vi "GetQR_A.vi"(8 "error in":errorcluster, 10 "Image In":T2, 11 "Session In":T1) -> (0 "error out":errorcluster, 1 "QR_OK":bool, 2 "QR_CODE":string, 3 "Image Out":T2(plugin-control))   [LabVIEW 2018]
uses:
  <vilib>/vision/Image Controls.llb/IMAQ Image.ctl
  <vilib>/userdefined/High Color/IMAQdx.ctl
  <vilib>/vision/NI_Vision_Development_Module.lvlib
  <vilib>/vision/driver/NI_Vision_Acquisition_Software.lvlib
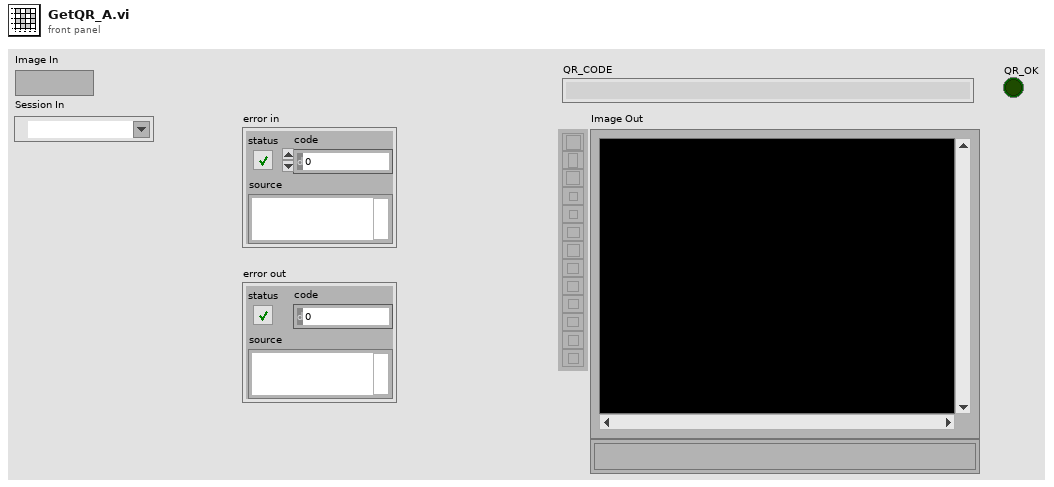
[diagram p1: front panel]
types:
  T1 = typedef "IMAQdx.ctl" = refnum<k21>
  T2 = typedef "IMAQ Image.ctl" = refnum<image>
  T3 = cluster{"Matrix Dimensions (cells)":i32, "Barcode Polarity":i32, "Mirror Mode":i32, "QR Model":i32}
  T4 = cluster{"Global Rectangle":i32[], "Contours":cluster{"ID":enum32{"External", "Internal"}, "Type":u32, "Coordinates":i32[]}[]}
  T5 = cluster{"Rotation Mode":enum32{"Unlimited", "0 Degrees", "90 Degrees", "180 Degrees", "270 Degrees"}, "Skip Location?":bool, "Edge Threshold":u32, "Demodulation Mode":i32, "Cell Sample Size":i32, "Cell Filter Mode":i32, "Skew Degrees Allowed":u32}
  T6 = typedef "QR Code Report.ctl" = cluster{"Found?":bool, "Data":string, "Bounding Box":cluster{"x":sgl, "y":sgl}[], "Errors Corrected":u32, "Dimensions (Rows/Cols)":u32, "Version":u32, "QR Model":T7, "Stream Mode":T8, "Barcode Polarity":T9, "Mirrored?":bool, "Append Stream Position":u32, "Size of Append Stream":u32, "First EAN-128 ID":i32, "First Alternate Language ID":i32, "Append Stream ID":u32, "Minimum Edge Strength":u32, "Demodulation Mode":T10, "Cell Sample Size":T11, "Cell Filter Mode":T12}
  T7 = typedef "QR Code Model Type.ctl" = i32
  T8 = typedef "QR Code Stream Mode Type.ctl" = i32
  T9 = typedef "Data Matrix Polarity.ctl" = i32
  T10 = typedef "Demodulation Mode.ctl" = i32
  T11 = typedef "Cell Sample Size.ctl" = i32
  T12 = typedef "Cell Filter Mode.ctl" = i32
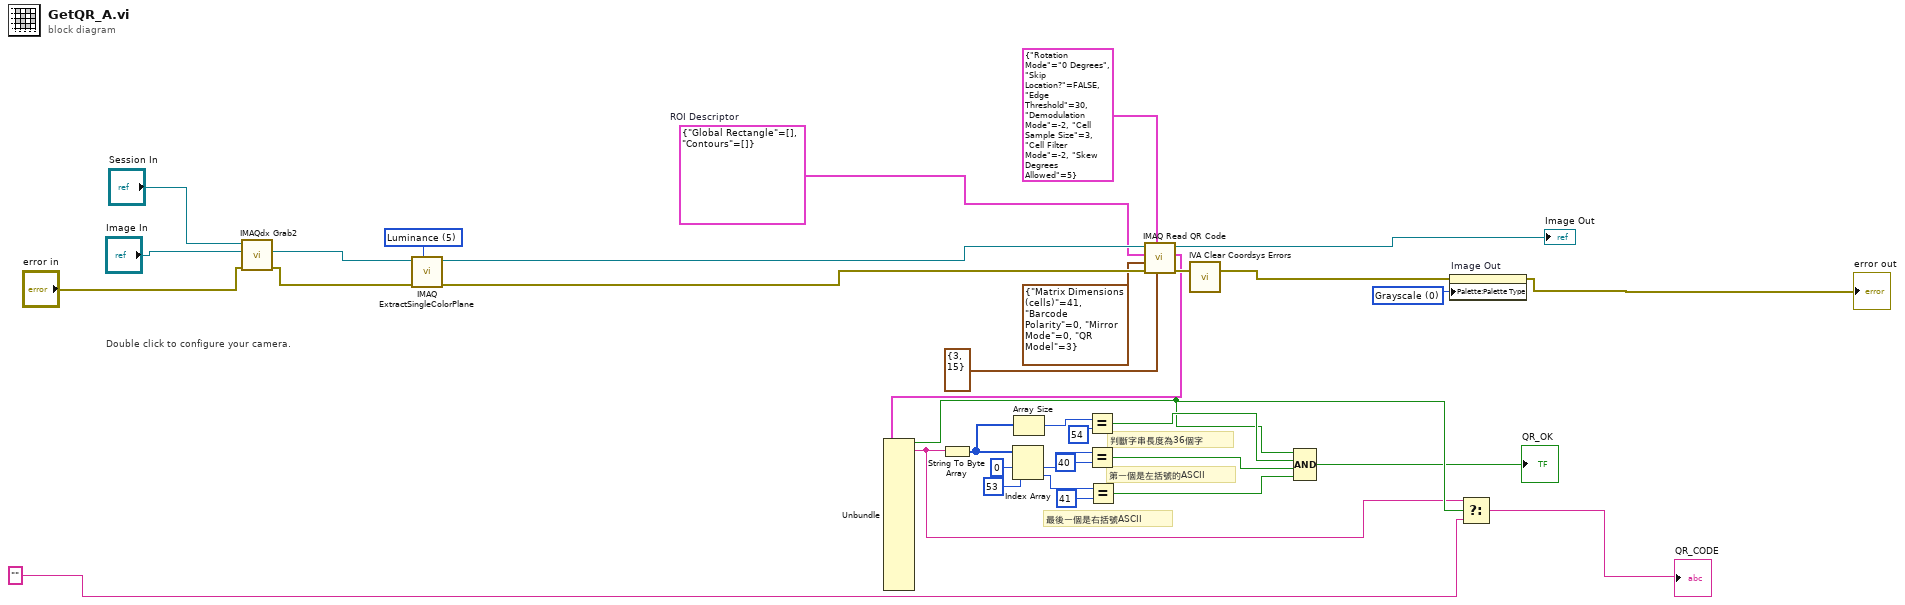
[diagram p0: block diagram]
diagram:
  w21 = u32 0 items=["Grayscale", "Binary", "Gradient", "Rainbow", "Temperature", "User Defined", "Binary 16 Bit", "Gradient 16 Bit", "Rainbow 16 Bit", "Temperature 16 Bit", "User Defined 16 Bit"] ("Palette Type")
  w25 = T4 {"Global Rectangle"=[], "Contours"=[]}  # ROI Descriptor
  w31 = 5 items=["Red", "Green", "Blue", "Hue", "Saturation", "Luminance", "Value", "Intensity"] ("Color Plane")
  # "最後一個是右括號ASCII"
  # "第一個是左括號的ASCII"
  # "判斷字串長度為36個字"
  # "Double click to configure your camera."
  n1 = call <vilib>:"IMAQdx Grab2.vi"("error in"="error in", "Image In"="Image In", "Session In"="Session In") -> ("error out"=w3:errorcluster, "Image Out"=w1:T2)  [unwired: 5 in, 2 out]
  n2 = call "IMAQ ExtractSingleColorPlane"("Color Plane"=w31, "error in (no error)"=w3, "Image Src"=w1) -> ("error out"=w30:errorcluster, "Image Dst Out"=w29:T2)  [unwired: 1 in, 6 out]
  n3 = call "IMAQ Read QR Code"("QR Code Cell Size (pixels)"=cluster{"Minimum Size":u32, "Maximum Size":u32} {"Minimum Size"=3, "Maximum Size"=15}, "QR Search Options"=T5 {"Rotation Mode"=enum."0 Degrees", "Skip Location?"=FALSE, "Edge Threshold"=30, "Demodulation Mode"=-2, "Cell Sample Size"=3, "Cell Filter Mode"=-2, "Skew Degrees Allowed"=5}, "error in (no error)"=w30, "QR Description Options"=T3 {"Matrix Dimensions (cells)"=41, "Barcode Polarity"=0, "Mirror Mode"=0, "QR Model"=3}, "ROI Descriptor"=w25, "Image"=w29) -> ("error out"=w24:errorcluster, "QR Code Report"=w20:T6, "Image (duplicate)"=→"Image Out":T2)  [unwired: 1 in, 2 out]
  n4 = Unbundle(w20) -> ("Found?"=w7:bool, "Data"=w6:string)  [unwired: 17 out]
  n5 = String To Byte Array(string=w6) -> (unsigned byte array=w8:u8[])
  n6 = Index Array(array=w8, index #1=0 ("index"), index #2=53 ("index")) -> (element #1=w15:u8, element #2=w14:u8)
  n7 = Array Size(array=w8) -> (size(s)=w19:i32)
  n8 = Equal?(x=w19, y=54) -> (x = y?=w11:bool)
  n9 = Equal?(x=w15, y=u8 40) -> (x = y?=w10:bool)
  n10 = Equal?(x=w14, y=u8 41) -> (x = y?=w9:bool)
  n11 = call <vilib>:"IVA Clear Coordsys Errors.vi"("error in (no error)"=w24) -> ("error out"=w23:errorcluster)  [unwired: 10 in]
  n12 = Compound Arithmetic op=AND(w7, w11, w10, w9) -> (→"QR_OK":bool)
  n13 = property on="Image Out" class="ImageControl"(error in=w23, "Palette:Palette Type"=w21) -> (error out=→"error out":errorcluster)  [unwired: 1 in, 1 out]
  n14 = Select(t=w6, s=w7, f="") -> (s? t:f=→"QR_CODE":string)
